vi "Actor Core.vi"(8 "error in":errorcluster, 11 "newport_xps in":refnum<class "newport_xps_panel.lvclass">) -> (0 "error out":errorcluster, 3 "Actor out":refnum<class "Actor.lvclass">)   [LabVIEW 2015, in "newport_xps_panel.lvclass"]
doc: "(<B>Filename</B>: Actor Framework.lvlib:Actor.lvclass:Actor Core.vi)\n\nReceives messages to the actor, reacts to them, and initiates any error handling that may shut the actor down.\n\nDescendant classes may override this VI to append parallel tasks for the actor to complete while it handles messages. Overrides use the Call Parent Method node."
uses:
  newport_xps_panel.lvclass
  <vilib>/ActorFramework/Actor/Actor.lvclass
  xps_login_info.ctl
  xps_actions.ctl
  newport_xps/dither_trajectory_settings.ctl
  newport_xps/dither_trajectory_types.ctl
  xps_panel_references.ctl
  newport_xps/newport_xps.lvclass
  UI/panel_class/panel.lvclass/panel.ctl
  newport_xps_panel.lvclass/newport_xps_panel.ctl
  <vilib>/ActorFramework/Actor/Actor.lvclass/Actor.ctl
  <vilib>/ActorFramework/Message Enqueuer/Message Enqueuer.lvclass/Message Enqueuer.ctl
  newport_xps_panel Messages/set_active_stage Msg/set_active_stage Msg.lvclass/set_active_stage Msg.ctl
  newport_xps_panel Messages/xps_panel_set_stage_speed Msg/xps_panel_set_stage_speed Msg.lvclass/xps_panel_set_stage_speed Msg.ctl
  newport_xps_panel Messages/xps_panel_move_stage_relative Msg/xps_panel_move_stage_relative Msg.lvclass/xps_panel_move_stage_relative Msg.ctl
  newport_xps_panel Messages/perform_stage_action Msg/perform_stage_action Msg.lvclass/perform_stage_action Msg.ctl
  newport_xps_panel Messages/xps_panel_generate_pvt_trajectory Msg/xps_panel_generate_pvt_trajectory Msg.lvclass/xps_panel_generate_pvt_trajectory Msg.ctl
  newport_xps_panel Messages/xps_panel_move_stage_absolute Msg/xps_panel_move_stage_absolute Msg.lvclass/xps_panel_move_stage_absolute Msg.ctl
  newport_xps_panel Messages/connect_to_controller Msg/connect_to_controller Msg.lvclass/connect_to_controller Msg.ctl
  <vilib>/ActorFramework/Message Enqueuer/Init from Existing Queue.vi
  <vilib>/ActorFramework/Message Enqueuer/Enqueue.vi
  <vilib>/ActorFramework/Message Priority Queue/Priority Enqueue.vi
  <vilib>/ActorFramework/Message Enqueuer/Message Enqueuer.lvclass
  newport_xps_panel Messages/set_active_stage Msg/set_active_stage Msg.lvclass
  newport_xps_panel Messages/xps_panel_set_stage_speed Msg/xps_panel_set_stage_speed Msg.lvclass
  newport_xps_panel Messages/xps_panel_move_stage_relative Msg/xps_panel_move_stage_relative Msg.lvclass
  newport_xps_panel Messages/perform_stage_action Msg/perform_stage_action Msg.lvclass
  newport_xps_panel Messages/xps_panel_generate_pvt_trajectory Msg/xps_panel_generate_pvt_trajectory Msg.lvclass
  newport_xps_panel Messages/xps_panel_dither_stage Msg/xps_panel_dither_stage Msg.lvclass
  newport_xps_panel Messages/xps_panel_move_stage_absolute Msg/xps_panel_move_stage_absolute Msg.lvclass
  newport_xps_panel Messages/xps_panel_retrive_ftp_trajectories Msg/xps_panel_retrive_ftp_trajectories Msg.lvclass
  newport_xps_panel Messages/connect_to_controller Msg/connect_to_controller Msg.lvclass
  newport_xps_panel Messages/disconnect_from_controller Msg/disconnect_from_controller Msg.lvclass
  UI/panel_class/panel.lvclass
panel:
  out "xps_position":dbl(graph) caption="Position mm"
  out "Status":string
  in  "controls":enum32{"Simple Movement", "Dither"}(tab)
  in  "abort_move":bool
  in  "jog_down":bool
  in  "jog_up":bool
  in  "Increment":dbl
  in  "move_absolute":bool
  in  "New Position":dbl
  in  "Speed":dbl=10.0
  out "current_position":dbl
  in  "stage_action":bool
  in  "Actions":T1
  in  "disconnect":bool
  in  "Login Info":T2={"IP Address"="192.168.0.254", "User"="Administrator", "Password"="Administrator"}
  in  "Stages":string(combo)
  in  "connect":bool
  in  "Chart Position":bool
  in  "Dither Cycles":u32=1
  in  "make_trajectory":bool
  in  "commence_dither":bool
  in  "Custom Dither Trajectory":T3={"PVT Ampl (nm)"=500.0, "Dither Period (s)"=10.0, "Type"=enum."Sawtooth", "Name"=""} {"Dither Period (s)" min=0.0; "PVT Ampl (nm)" min=0.0}
  in  "retrieve_trajectories":bool
  in  "Select Trajectory":string(combo)
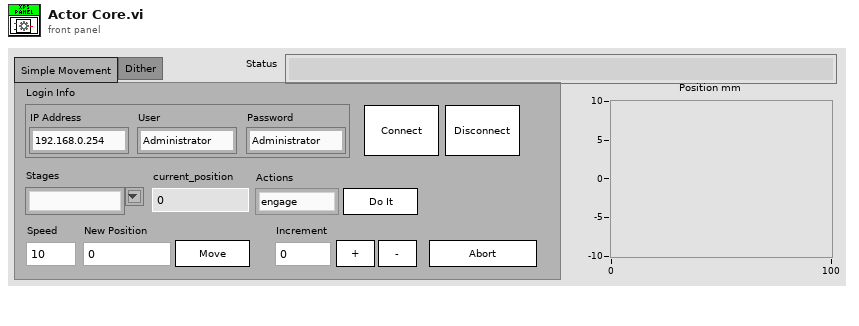
[diagram p1: front panel]
types:
  T1 = typedef "xps_actions.ctl" = enum16{"engage", "home", "kill"}
  T2 = typedef "xps_login_info.ctl" = cluster{"IP Address":string, "User":string, "Password":string}
  T3 = typedef "dither_trajectory_settings.ctl" = cluster{"PVT Ampl (nm)":dbl, "Dither Period (s)":dbl, "Type":T4, "Name":string}
  T4 = typedef "dither_trajectory_types.ctl" = enum16{"Sawtooth"}
  T5 = typedef "xps_panel_references.ctl" = cluster{"xps_position_chart":refnum<vi>, "Status":refnum<vi>, "current_position":refnum<vi>, "Stages":refnum<vi>}
  T6 = typedef "event_references.ctl" = cluster{"update_position":refnum<event-registration>, "abort_move":refnum<event-registration>, "update_xps_status":refnum<event-registration>, "retrieve_trajectories":refnum<event-registration>, "set_available_stages":refnum<event-registration>}
  T7 = cluster{"update_position":refnum<event-registration>, "stop_ui_ref":refnum<event-registration>, "update_xps_status":refnum<event-registration>, "retrieve_trajectories":refnum<event-registration>, "set_available_stages":refnum<event-registration>}
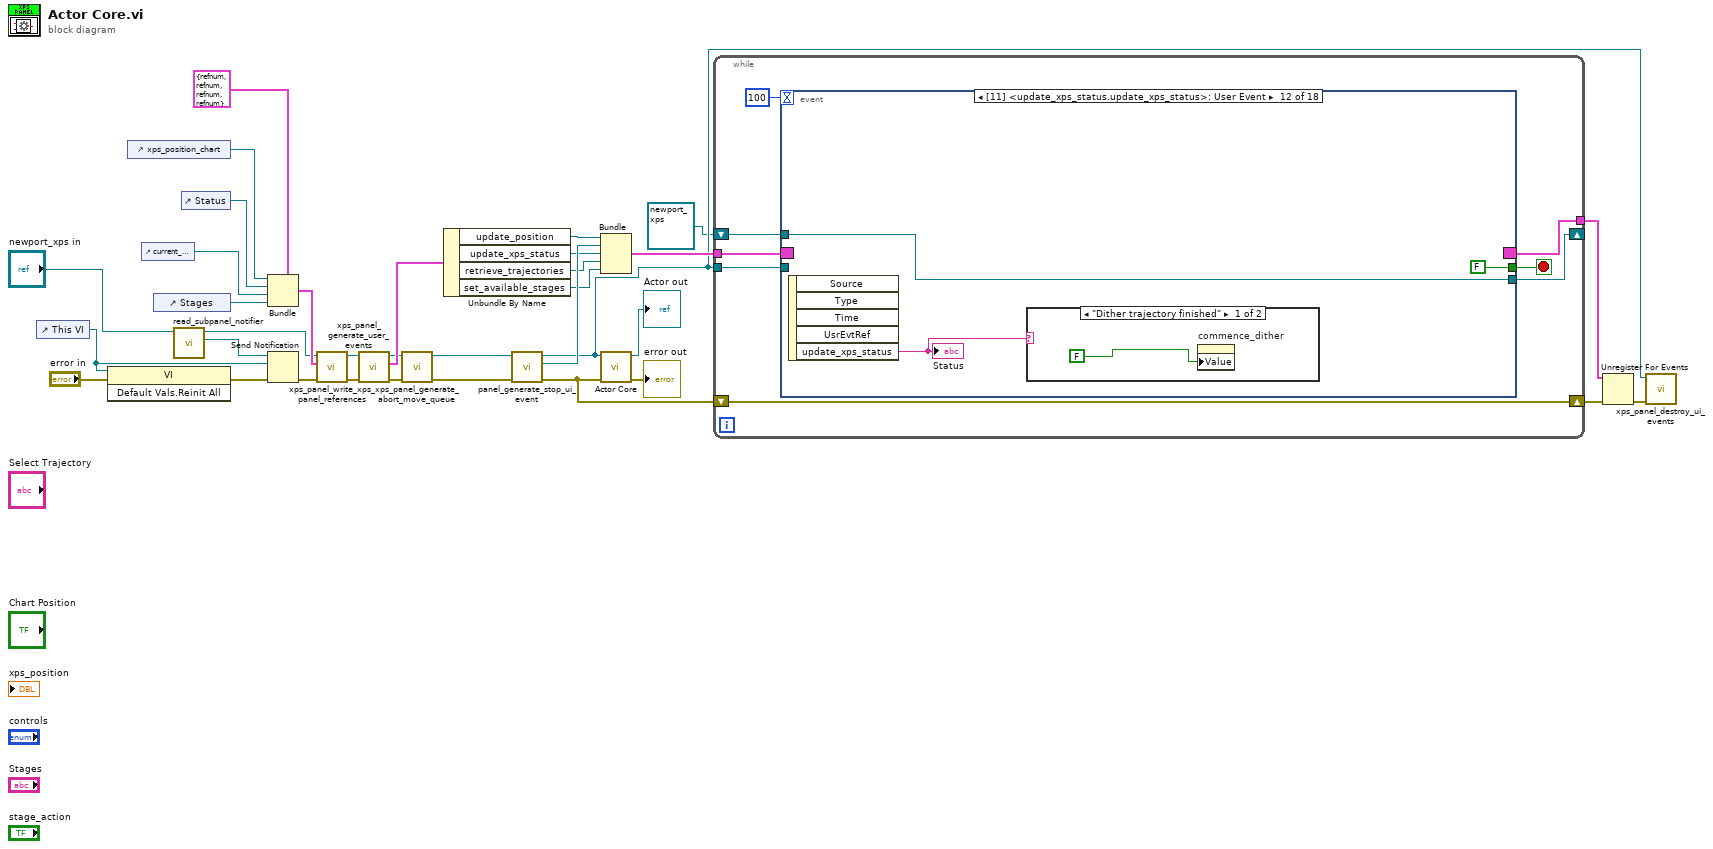
[diagram p0: block diagram]
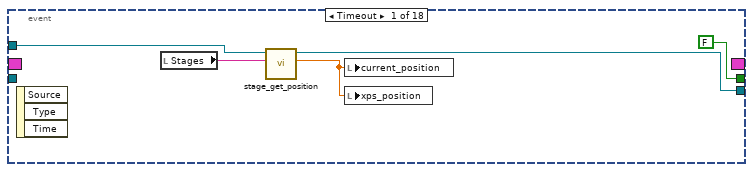
[diagram p2: hidden frame]
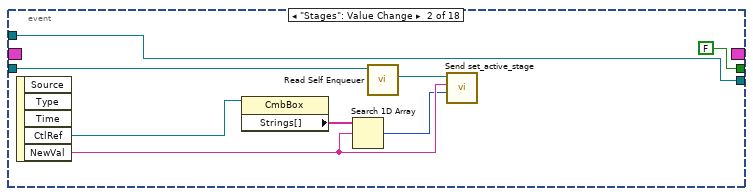
[diagram p3: hidden frame]
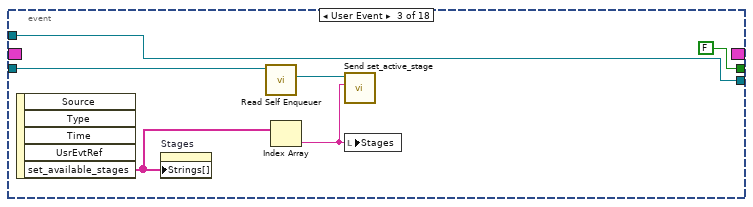
[diagram p4: hidden frame]
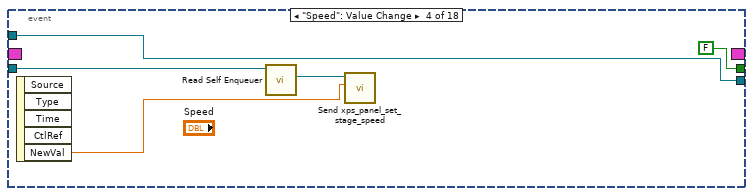
[diagram p5: hidden frame]
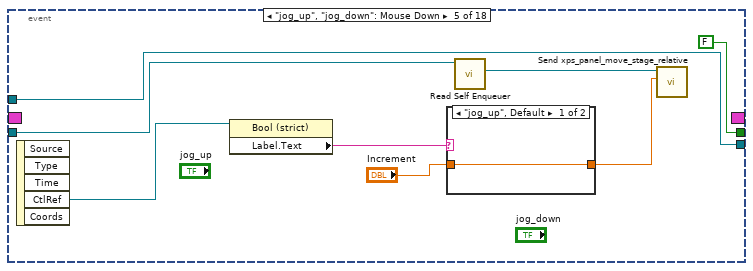
[diagram p6: hidden frame]
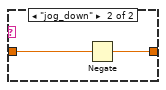
[diagram p7: hidden frame]
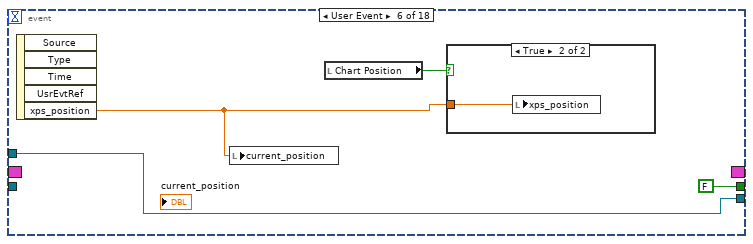
[diagram p8: hidden frame]
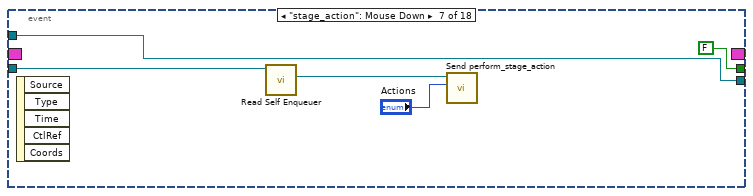
[diagram p10: hidden frame]
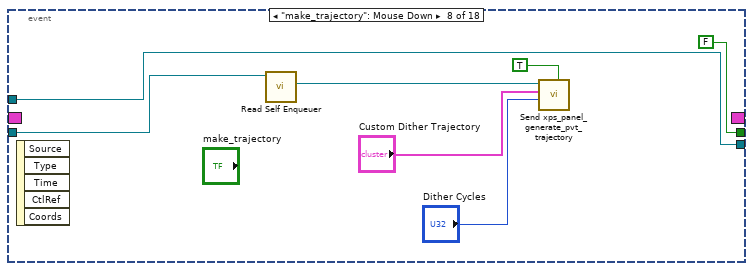
[diagram p11: hidden frame]
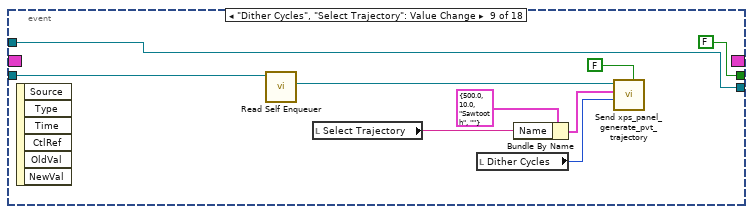
[diagram p12: hidden frame]
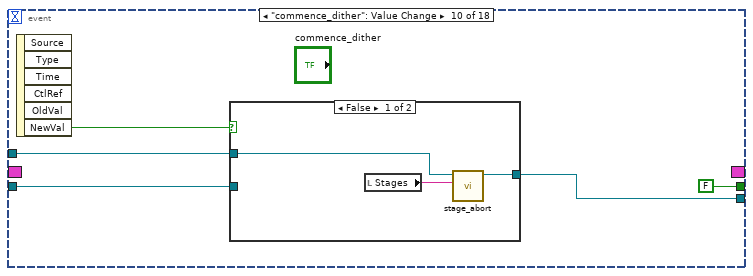
[diagram p13: hidden frame]
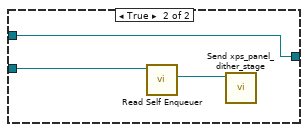
[diagram p14: hidden frame]
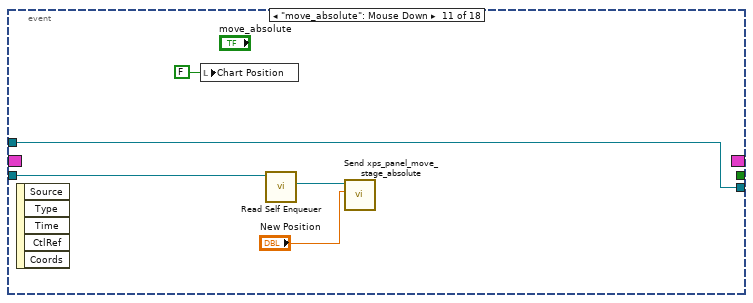
[diagram p15: hidden frame]
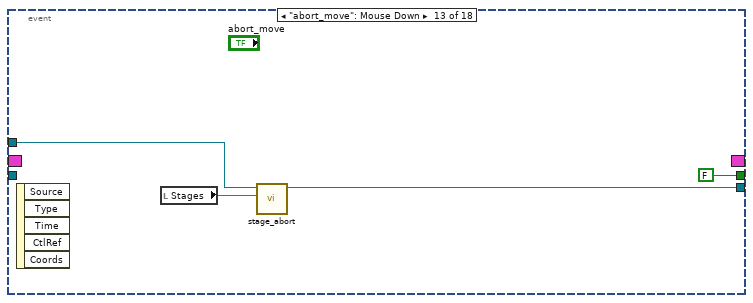
[diagram p17: hidden frame]
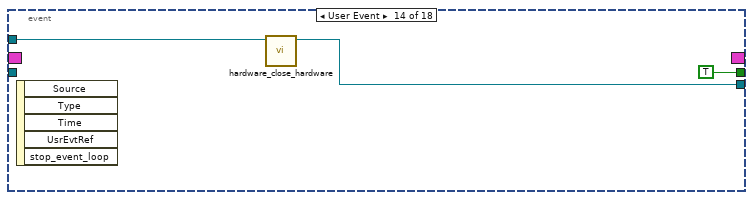
[diagram p18: hidden frame]
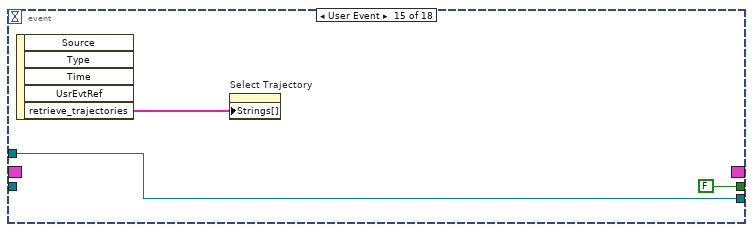
[diagram p19: hidden frame]
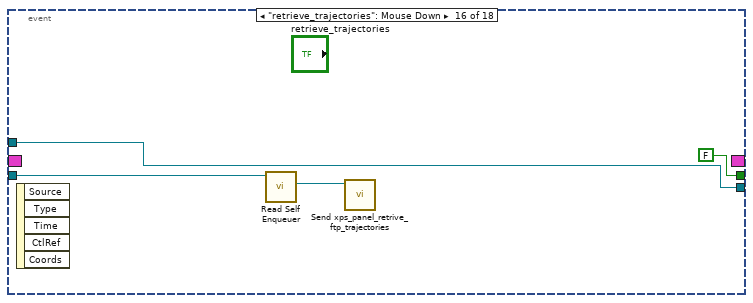
[diagram p20: hidden frame]
diagram:
  n1 = control-ref of="This VI"() -> (w22:refnum<vi>)
  n2 = invoke class="VI" method="Default Vals.Reinit All"(reference=w22, error in="error in") -> (error out=w11:errorcluster)  [unwired: 1 in, 2 out]
  n3 = control-ref of="xps_position_chart"() -> (w29:refnum<vi>)
  n4 = control-ref of="current_position"() -> (w27:refnum<vi>)
  n5 = control-ref of="Stages"() -> (w23:refnum<vi>)
  n6 = call "read_subpanel_notifier.vi"("panel in"="newport_xps in") -> ("subpanel_notifier"=w15:refnum<notifier>, "panel out"=w13:refnum<class "newport_xps_panel.lvclass">)  [unwired: 8 in, 1 out]
  n7 = control-ref of="Status"() -> (w28:refnum<vi>)
  n8 = Bundle(cluster=T5 {"xps_position_chart"=refnum, "Status"=refnum, "current_position"=refnum, "Stages"=refnum} ("output cluster"), "xps_position_chart"=w29, "Status"=w28, "current_position"=w27, "Stages"=w23) -> (w24:T5)
  n9 = Send Notification(notification=w22, notifier=w15, error in (no error)=w11) -> (error out=w25:errorcluster)  [unwired: 1 out]
  n10 = call "xps_panel_write_xps_panel_references.vi"("error in (no error)"=w25, "xps_panel_references"=w24, "newport_xps_panel in"=w13) -> ("error out"=w21:errorcluster, "newport_xps_panel out"=w20:refnum<class "newport_xps_panel.lvclass">)  [unwired: 7 in]
  n11 = call "xps_panel_generate_user_events.vi"("error in (no error)"=w21, "newport_xps_panel in"=w20) -> ("error out"=w5:errorcluster, "event_references"=w19:T6, "newport_xps_panel out"=w8:refnum<class "newport_xps_panel.lvclass">)  [unwired: 7 in]
  n12 = call "xps_panel_generate_abort_move_queue.vi"("error in (no error)"=w5, "newport_xps_panel in"=w8) -> ("error out"=w6:errorcluster, "newport_xps_panel out"=w7:refnum<class "newport_xps_panel.lvclass">)  [unwired: 8 in]
  n13 = Unbundle By Name(w19) -> ("update_position"=w17:refnum<event-registration>, "update_xps_status"=w10:refnum<event-registration>, "retrieve_trajectories"=w9:refnum<event-registration>, "set_available_stages"=w1:refnum<event-registration>)
  n14 = call "panel_generate_stop_ui_event.vi"("error in (no error)"=w6, "panel in"=w7) -> ("error out"=w32:errorcluster, "stop_ui_ref"=w18:refnum<event-registration>, "panel out"=w3:refnum<class "newport_xps_panel.lvclass">)  [unwired: 7 in]
  n15 = Bundle("update_position"=w17, "stop_ui_ref"=w18, "update_xps_status"=w10, "retrieve_trajectories"=w9, "set_available_stages"=w1) -> (w16:T7)  [unwired: 1 in]
  n16 = call-parent "Actor Core.vi"("error in"=w32, "Actor in"=w3) -> ("error out"=→"error out":errorcluster, "Actor out"=→"Actor out":refnum<class "Actor.lvclass">)  [unwired: 8 in]
  n17 = while {
    tunnel: w16 -> [w42]
    shift-right: [w40] -> w31
    shift-left: w32 -> [w40]
    tunnel: [w39] -> w30
    tunnel: w3 -> [w37]
    shift-right: [w35] -> _
    shift-left: refnum<class "newport_xps.lvclass"> refnum ("newport_xps out") -> [w36]
    stop <- w41 stop-if-true
    n18 = event shown="[11] <update_xps_status.update_xps_status>: User Event" {
      selector: w42 -> [_ _ _ _ _ _ _ _ _ _ _ _ _ _ _ _ _ _]
      dyn-events: [_ _ _ _ _ _ _ _ _ _ _ _ _ _ _ _ _ _] -> w39
      timeout: 100 -> [_ _ _ _ _ _ _ _ _ _ _ _ _ _ _ _ _ _]
      tunnel: [FALSE FALSE FALSE FALSE FALSE FALSE FALSE FALSE FALSE FALSE _ FALSE FALSE TRUE FALSE FALSE FALSE FALSE] -> w41
      tunnel: w37 -> [_ w55 w58 w66 w72 _ w87 w94 w101 w107 w119 _ _ _ _ w137 w147 w153]
      tunnel: w36 -> [w46 w48 w60 w63 w67 w78 w83 w88 w96 w105 w115 w121 w126 w129 w131 w134 w145 w150]
      tunnel: [w43 w48 w60 w63 w67 w78 w83 w88 w96 w104 w115 w121 w125 w128 w131 w134 w138 w149] -> w35
      event Timeout {
        n19 = event-data() -> ()  [unwired: 1 in, 3 out]
        n20 = local read "Stages"() -> (w44:string)
        n21 = call-dynamic "stage_get_position.vi"("Stage Name"=w44, "newport_xps in"=w46) -> ("Position"=w45:dbl, "newport_xps out"=w43:refnum<class "newport_xps.lvclass">)  [unwired: 7 in, 1 out]
        n22 = local write "current_position"(w45) -> ()
        n23 = local write "xps_position"(w45) -> ()
      }
      event "Stages": Value Change {
        n24 = event-data() -> ("CtlRef"=w53:refnum<vi>, "NewVal"=w51:string)  [unwired: 1 in, 3 out]
        n25 = property class="CmbBox"(reference=w53) -> ("Strings[]"=w52:string[])  [unwired: 1 in, 2 out]
        n26 = Search 1D Array(1D array=w52, element=w51) -> (index of element=w50:i32)  [unwired: 1 in]
        n27 = call <vilib>:"Read Self Enqueuer.vi"("Actor"=w55) -> ("Self Enqueuer"=w54:refnum<class "Message Enqueuer.lvclass">)  [unwired: 10 in]
        n28 = call "Send set_active_stage.vi"("stage_number"=w50, "stage_name"=w51, "Message Enqueuer"=w54) -> ()  [unwired: 7 in, 2 out]
      }
      event User Event {
        n29 = event-data() -> ("set_available_stages"=w61:string[])  [unwired: 1 in, 4 out]
        n30 = property on="Stages" class="CmbBox"("Strings[]"=w61) -> ()  [unwired: 2 in, 2 out]
        n31 = call <vilib>:"Read Self Enqueuer.vi"("Actor"=w58) -> ("Self Enqueuer"=w57:refnum<class "Message Enqueuer.lvclass">)  [unwired: 10 in]
        n32 = Index Array(array=w61) -> (element=w56:string)  [unwired: 1 in]
        n33 = call "Send set_active_stage.vi"("stage_name"=w56, "Message Enqueuer"=w57) -> ()  [unwired: 8 in, 2 out]
        n34 = local write "Stages"(w56) -> ()
      }
      event "Speed": Value Change {
        n35 = event-data() -> ("NewVal"=w64:dbl)  [unwired: 1 in, 4 out]
        n36 = call <vilib>:"Read Self Enqueuer.vi"("Actor"=w66) -> ("Self Enqueuer"=w65:refnum<class "Message Enqueuer.lvclass">)  [unwired: 10 in]
        n37 = call "Send xps_panel_set_stage_speed.vi"("stage_speed"=w64, "Message Enqueuer"=w65) -> ()  [unwired: 8 in, 2 out]
      }
      event "jog_up", "jog_down": Mouse Down {
        n38 = event-data() -> ("CtlRef"=w74:refnum<vi>)  [unwired: 1 in, 4 out]
        n39 = property class="Bool (strict)"(reference=w74) -> ("Label.Text"=w73:string)  [unwired: 1 in, 2 out]
        n40 = case shown="\"jog_up\", Default" w73 {
          tunnel: "Increment" -> [w75 w77]
          tunnel: [w75 w76] -> w69
          frame "jog_up", Default {
          }
          frame "jog_down" {
            n41 = Negate(x=w77) -> (-x=w76:dbl)
          }
        }
        n42 = call <vilib>:"Read Self Enqueuer.vi"("Actor"=w72) -> ("Self Enqueuer"=w70:refnum<class "Message Enqueuer.lvclass">)  [unwired: 10 in]
        n43 = call "Send xps_panel_move_stage_relative.vi"("displacement"=w69, "Message Enqueuer"=w70) -> ()  [unwired: 8 in, 2 out]
      }
      event User Event {
        n44 = event-data() -> ("xps_position"=w80:dbl)  [unwired: 1 in, 4 out]
        n45 = local write "current_position"(w80) -> ()
        n46 = local read "Chart Position"() -> (w81:bool)
        n47 = case shown="True" w81 {
          tunnel: w80 -> [_ w82]
          frame False {
          }
          frame True {
            n48 = local write "xps_position"(w82) -> ()
          }
        }
      }
      event "stage_action": Mouse Down {
        n49 = event-data() -> ()  [unwired: 1 in, 5 out]
        n50 = call <vilib>:"Read Self Enqueuer.vi"("Actor"=w87) -> ("Self Enqueuer"=w86:refnum<class "Message Enqueuer.lvclass">)  [unwired: 10 in]
        n51 = call "Send perform_stage_action.vi"("xps_actions"="Actions", "Message Enqueuer"=w86) -> ()  [unwired: 8 in, 2 out]
      }
      event "make_trajectory": Mouse Down {
        n52 = event-data() -> ()  [unwired: 1 in, 5 out]
        n53 = call <vilib>:"Read Self Enqueuer.vi"("Actor"=w94) -> ("Self Enqueuer"=w93:refnum<class "Message Enqueuer.lvclass">)  [unwired: 10 in]
        n54 = call "Send xps_panel_generate_pvt_trajectory.vi"("custom?"=TRUE, "Dither Cycles"="Dither Cycles", "Custom Dither Trajectory"="Custom Dither Trajectory", "Message Enqueuer"=w93) -> ()  [unwired: 6 in, 2 out]
      }
      event "Dither Cycles", "Select Trajectory": Value Change {
        n55 = event-data() -> ()  [unwired: 1 in, 6 out]
        n56 = call <vilib>:"Read Self Enqueuer.vi"("Actor"=w101) -> ("Self Enqueuer"=w103:refnum<class "Message Enqueuer.lvclass">)  [unwired: 10 in]
        n57 = local read "Select Trajectory"() -> (w97:string)
        n58 = local read "Dither Cycles"() -> (w98:u32)
        n59 = Bundle By Name(cluster=T3 {"PVT Ampl (nm)"=500.0, "Dither Period (s)"=10.0, "Type"=enum."Sawtooth", "Name"=""} ("Custom Dither Trajectory"), "Name"=w97) -> (w99:T3)
        n60 = call "Send xps_panel_generate_pvt_trajectory.vi"("custom?"=FALSE, "Dither Cycles"=w98, "Custom Dither Trajectory"=w99, "Message Enqueuer"=w103) -> ()  [unwired: 6 in, 2 out]
      }
      event "commence_dither": Value Change {
        n61 = event-data() -> ("NewVal"=w108:bool)  [unwired: 1 in, 5 out]
        n62 = case shown="False" w108 {
          tunnel: w107 -> [_ w114]
          tunnel: w105 -> [w111 w112]
          tunnel: [w110 w112] -> w104
          frame False {
            n63 = local read "Stages"() -> (w109:string)
            n64 = call-dynamic "stage_abort.vi"("Stage Name"=w109, "newport_xps in"=w111) -> ("newport_xps out"=w110:refnum<class "newport_xps.lvclass">)  [unwired: 8 in, 1 out]
          }
          frame True {
            n65 = call <vilib>:"Read Self Enqueuer.vi"("Actor"=w114) -> ("Self Enqueuer"=w113:refnum<class "Message Enqueuer.lvclass">)  [unwired: 10 in]
            n66 = call "Send xps_panel_dither_stage.vi"("Message Enqueuer"=w113) -> ()  [unwired: 9 in, 2 out]
          }
        }
      }
      event "move_absolute": Mouse Down {
        n67 = event-data() -> ()  [unwired: 1 in, 5 out]
        n68 = local write "Chart Position"(FALSE ("Chart Position")) -> ()
        n69 = call <vilib>:"Read Self Enqueuer.vi"("Actor"=w119) -> ("Self Enqueuer"=w118:refnum<class "Message Enqueuer.lvclass">)  [unwired: 10 in]
        n70 = call "Send xps_panel_move_stage_absolute.vi"("Position"="New Position", "Message Enqueuer"=w118) -> ()  [unwired: 8 in, 2 out]
      }
      event User Event {
        n71 = event-data() -> ("update_xps_status"=w120:string)  [unwired: 1 in, 4 out]
        "Status" <- w120
        n72 = case shown="\"Dither trajectory finished\"" w120 {
          frame "Dither trajectory finished" {
            n73 = property on="commence_dither" class="Bool (strict)"("Value"=FALSE ("commence_dither")) -> ()  [unwired: 2 in, 2 out]
          }
          frame Default {
          }
        }
      }
      event "abort_move": Mouse Down {
        n74 = event-data() -> ()  [unwired: 1 in, 5 out]
        n75 = local read "Stages"() -> (w124:string)
        n76 = call-dynamic "stage_abort.vi"("Stage Name"=w124, "newport_xps in"=w126) -> ("newport_xps out"=w125:refnum<class "newport_xps.lvclass">)  [unwired: 8 in, 1 out]
      }
      event User Event {
        n77 = event-data() -> ()  [unwired: 1 in, 5 out]
        n78 = call-dynamic "hardware_close_hardware.vi"("newport_xps in"=w129) -> ("newport_xps out"=w128:refnum<class "newport_xps.lvclass">)  [unwired: 9 in, 1 out]
      }
      event User Event {
        n79 = event-data() -> ("retrieve_trajectories"=w133:string[])  [unwired: 1 in, 4 out]
        n80 = property on="Select Trajectory" class="CmbBox"("Strings[]"=w133) -> ()  [unwired: 2 in, 2 out]
      }
      event "retrieve_trajectories": Mouse Down {
        n81 = event-data() -> ()  [unwired: 1 in, 5 out]
        n82 = call <vilib>:"Read Self Enqueuer.vi"("Actor"=w137) -> ("Self Enqueuer"=w136:refnum<class "Message Enqueuer.lvclass">)  [unwired: 10 in]
        n83 = call "Send xps_panel_retrive_ftp_trajectories.vi"("Message Enqueuer"=w136) -> ()  [unwired: 9 in, 2 out]
      }
      event "connect": Mouse Down {
        n84 = event-data() -> ()  [unwired: 1 in, 5 out]
        n85 = call <vilib>:"Read Self Enqueuer.vi"("Actor"=w147) -> ("Self Enqueuer"=w146:refnum<class "Message Enqueuer.lvclass">)  [unwired: 10 in]
        n86 = call "Send connect_to_controller.vi"("Login Info"="Login Info", "Message Enqueuer"=w146) -> ()  [unwired: 8 in, 2 out]
        n87 = Unbundle By Name("Login Info") -> ("IP Address"=w143:string, "User"=w142:string, "Password"=w141:string)
        n88 = call "write_login_info.vi"("IP address"=w143, "Password"=w141, "User"=w142, "newport_xps in"=w145) -> ("error out"=w140:errorcluster, "newport_xps out"=w139:refnum<class "newport_xps.lvclass">)  [unwired: 6 in]
        n89 = call-dynamic "hardware_initialize_hardware.vi"("error in (no error)"=w140, "newport_xps in"=w139) -> ("newport_xps out"=w138:refnum<class "newport_xps.lvclass">)  [unwired: 8 in, 1 out]
      }
      event "disconnect": Mouse Down {
        n90 = event-data() -> ()  [unwired: 1 in, 5 out]
        n91 = call <vilib>:"Read Self Enqueuer.vi"("Actor"=w153) -> ("Self Enqueuer"=w152:refnum<class "Message Enqueuer.lvclass">)  [unwired: 10 in]
        n92 = call "Send disconnect_from_controller.vi"("Message Enqueuer"=w152) -> ()  [unwired: 9 in, 2 out]
        n93 = call-dynamic "hardware_close_hardware.vi"("newport_xps in"=w150) -> ("newport_xps out"=w149:refnum<class "newport_xps.lvclass">)  [unwired: 9 in, 1 out]
      }
    }
  }
  n94 = Unregister For Events(event registration refnum=w30, error in=w31) -> (error out=w4:errorcluster)
  n95 = call "xps_panel_destroy_ui_events.vi"("error in (no error)"=w4, "newport_xps_panel in"=w3) -> ()  [unwired: 8 in, 2 out]
